vi "TuneFreq.vi"(0 "SG GPIB Address":dbl=22.0, 1 "Trigger Delay":dbl=59.0, 2 "Mod Freq (Hz)":dbl=47.0, 3 "Amplitude (V)":dbl=1.0, 4 "Burst count":dbl=205.0, 5 "PS GPIB Address":string="1", 7 "Poly Coeffs":dbl[](array[numeric]), 9 "Field Set (Oe)":dbl, 11 "VNA GPIB Address":refnum<visa-resource-name>="GPIB0::15::INSTR", 12 "IF Bandwidth":dbl=1000.0, 13 "VNA Points":dbl=1000.0, 14 "VNA Frequency":dbl=10.0, 15 "VNA Power (dBm)":string="-10") -> (8 "Re Freq":dbl format="%.4f")   [LabVIEW 2015]
uses:
  <vilib>/Utility/file.llb/Read Delimited Spreadsheet (DBL).vi
panel:
  out "Im Freq":dbl format="%.4f"
  out "Phase":dbl[][](graph)
  out "Amplitude":dbl[][](graph)
  out "Re phase (deg)":dbl format="%.3f"
  out "Re amplitude":dbl format="%.2e"
  out "Im phase (deg)":dbl format="%.3f"
  out "Im amplitude":dbl format="%.2e"
  out "Im VNA Output":cluster{"X-values":dbl[], "Input data":dbl[]}[](graph)
  out "Re VNA Output":cluster{"X-values":dbl[], "Input data":dbl[]}[](graph)
  in  "Done":bool
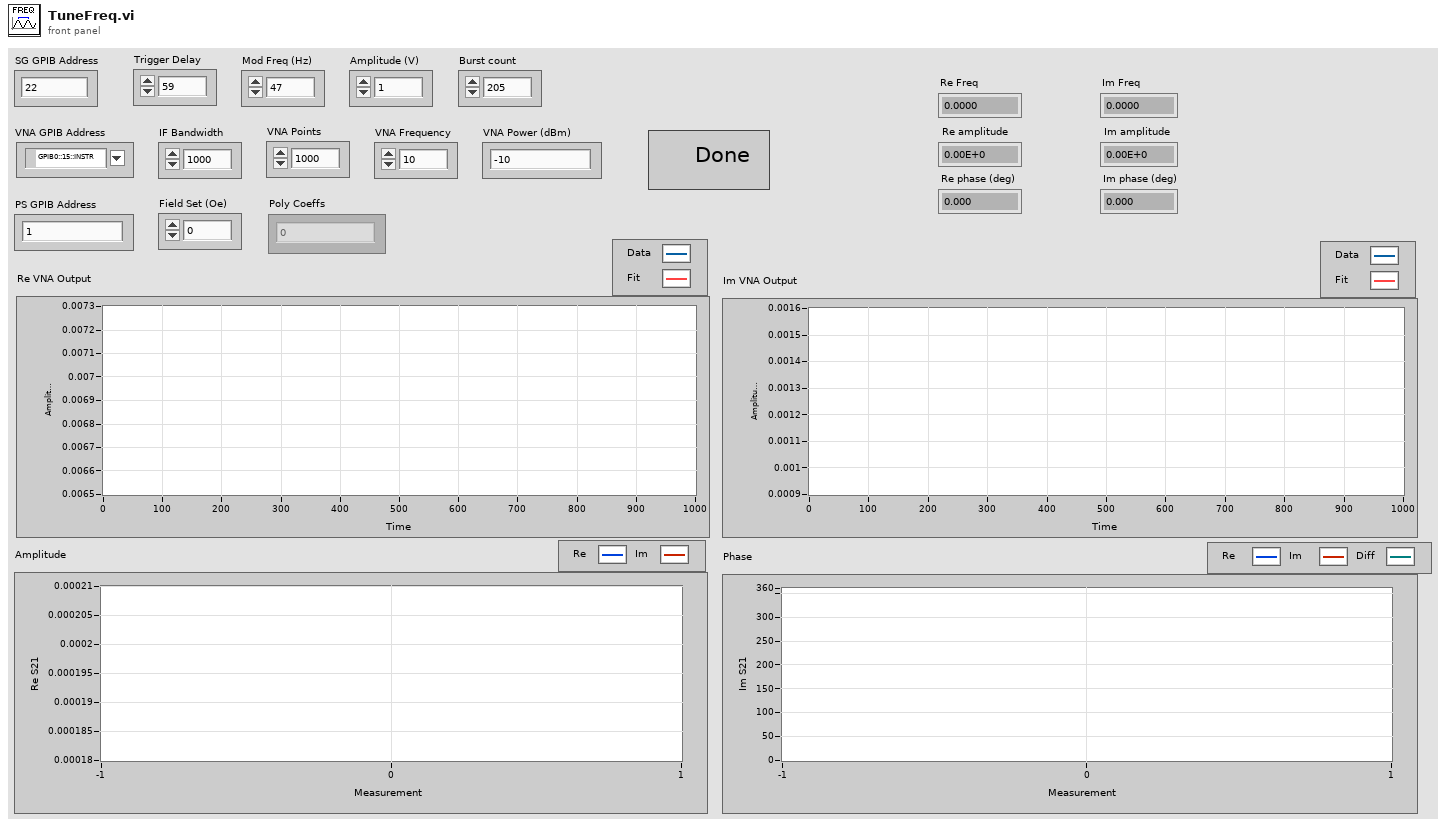
[diagram p1: front panel]
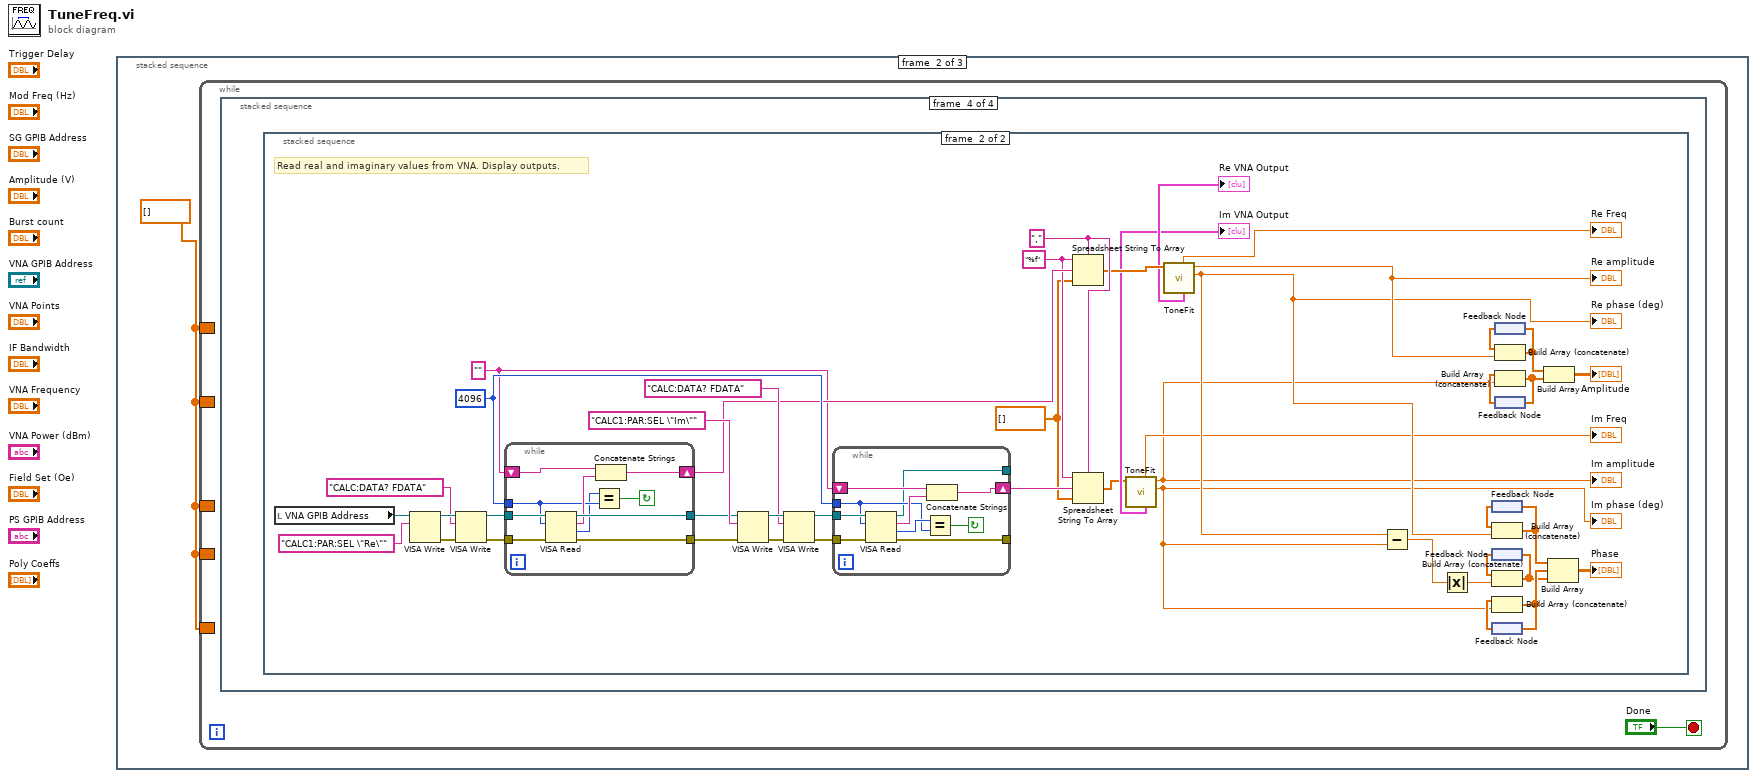
[diagram p0: block diagram]
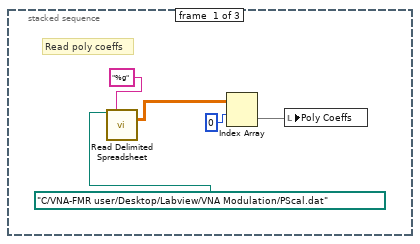
[diagram p2: hidden frame]
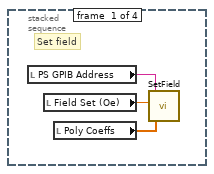
[diagram p3: hidden frame]
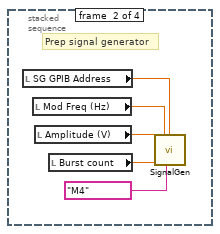
[diagram p4: hidden frame]
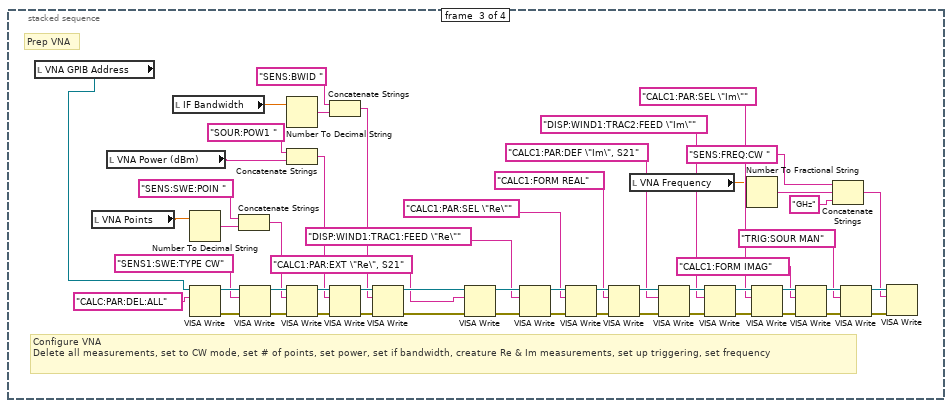
[diagram p5: hidden frame]
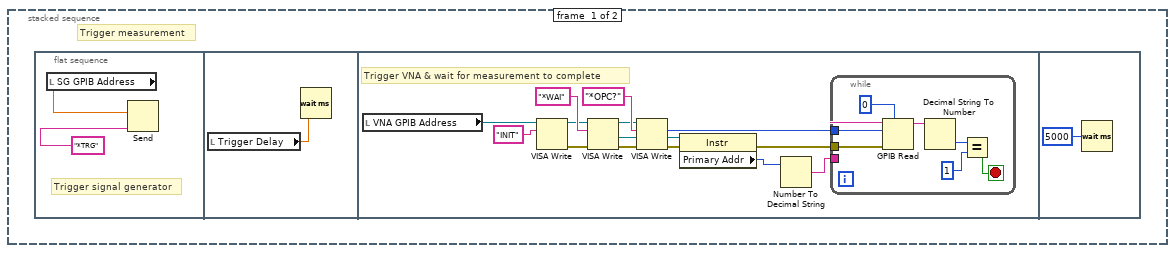
[diagram p6: hidden frame]
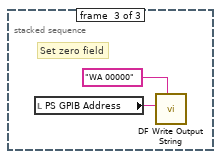
[diagram p7: hidden frame]
diagram:
  n1 = stacked-sequence {
    frame #0 {
      # "Read poly coeffs"
      n2 = call-poly <vilib>:"Read Delimited Spreadsheet.vi"("file path (dialog if empty)"=path "C:/VNA-FMR user/Desktop/Labview/VNA Modulation/PScal.dat", "format (%.3f)"="%g") -> ("all rows"=w3:dbl[][])  [unwired: 8 in, 5 out]
      n3 = Index Array(array=w3, index (row)=0 ("disabled index (col)")) -> (element=w1:dbl[])  [unwired: 1 in]
      n4 = local write "Poly Coeffs"(w1) -> ()
    }
    frame #1 {
      w6 = dbl[] []
      n5 = while {
        border: w6 -> [_]
        border: w6 -> [_]
        border: w6 -> [_]
        border: w6 -> [_]
        border: w6 -> [_]
        stop <- "Done" stop-if-true
        n6 = stacked-sequence {
          frame #0 {
            # "Set field"
            n7 = local read "PS GPIB Address"() -> (w10:string)
            n8 = local read "Field Set (Oe)"() -> (w9:dbl)
            n9 = local read "Poly Coeffs"() -> (w8:dbl[])
            n10 = call "SetField.vi"("Poly Coeffs"=w8, "Field Setpoint"=w9, "PS GPIB Address"=w10) -> ()  [unwired: 9 in]
          }
          frame #1 {
            # "Prep signal generator"
            n11 = local read "SG GPIB Address"() -> (w15:dbl)
            n12 = local read "Mod Freq (Hz)"() -> (w14:dbl)
            n13 = local read "Amplitude (V)"() -> (w13:dbl)
            n14 = local read "Burst count"() -> (w12:dbl)
            n15 = call "SignalGen.vi"("Trigger Mode (Cont)"="M4", "Burst Count"=w12, "Amplitide (V)"=w13, "Modulation Frequency (Hz)"=w14, "SG GPIB Address"=w15) -> ()  [unwired: 7 in]
          }
          frame #2 {
            # "Configure VNA\nDelete all measurements, set to CW mode, set # of points, set power, set if bandwidth, creature Re & Im measurements, set up triggering, set frequency"
            # "Prep VNA"
            n16 = local read "VNA GPIB Address"() -> (w20:refnum<visa-resource-name>)
            n17 = local read "VNA Points"() -> (w19:dbl)
            n18 = local read "VNA Power (dBm)"() -> (w18:string)
            n19 = local read "IF Bandwidth"() -> (w17:dbl)
            n20 = Number To Decimal String(number=w19) -> (decimal integer string=w66:string)  [unwired: 1 in]
            n21 = VISA Write(VISA resource name=w20, write buffer="CALC:PAR:DEL:ALL" ("Characters to Write")) -> (VISA resource name out=w71:refnum<visa-resource-name>, error out=w28:errorcluster)  [unwired: 1 in, 1 out]
            n22 = Concatenate Strings("SENS:SWE:POIN " ("Characters to Write"), w66) -> (w65:string)
            n23 = VISA Write(VISA resource name=w71, write buffer="SENS1:SWE:TYPE CW" ("Characters to Write"), error in (no error)=w28) -> (VISA resource name out=w68:refnum<visa-resource-name>, error out=w69:errorcluster)  [unwired: 1 out]
            n24 = Number To Decimal String(number=w17) -> (decimal integer string=w57:string)  [unwired: 1 in]
            n25 = Concatenate Strings("SOUR:POW1 " ("Characters to Write"), w18) -> (w61:string)
            n26 = VISA Write(VISA resource name=w68, write buffer=w65, error in (no error)=w69) -> (VISA resource name out=w63:refnum<visa-resource-name>, error out=w64:errorcluster)  [unwired: 1 out]
            n27 = Concatenate Strings("SENS:BWID " ("Characters to Write"), w57) -> (w56:string)
            n28 = VISA Write(VISA resource name=w63, write buffer=w61, error in (no error)=w64) -> (VISA resource name out=w59:refnum<visa-resource-name>, error out=w60:errorcluster)  [unwired: 1 out]
            n29 = VISA Write(VISA resource name=w59, write buffer=w56, error in (no error)=w60) -> (VISA resource name out=w54:refnum<visa-resource-name>, error out=w55:errorcluster)  [unwired: 1 out]
            n30 = VISA Write(VISA resource name=w54, write buffer="CALC1:PAR:EXT \"Re\", S21" ("Characters to Write"), error in (no error)=w55) -> (VISA resource name out=w51:refnum<visa-resource-name>, error out=w52:errorcluster)  [unwired: 1 out]
            n31 = VISA Write(VISA resource name=w51, write buffer="DISP:WIND1:TRAC1:FEED \"Re\"" ("Characters to Write"), error in (no error)=w52) -> (VISA resource name out=w48:refnum<visa-resource-name>, error out=w49:errorcluster)  [unwired: 1 out]
            n32 = VISA Write(VISA resource name=w48, write buffer="CALC1:PAR:SEL \"Re\"" ("Characters to Write"), error in (no error)=w49) -> (VISA resource name out=w45:refnum<visa-resource-name>, error out=w46:errorcluster)  [unwired: 1 out]
            n33 = VISA Write(VISA resource name=w45, write buffer="CALC1:FORM REAL" ("Characters to Write"), error in (no error)=w46) -> (VISA resource name out=w42:refnum<visa-resource-name>, error out=w43:errorcluster)  [unwired: 1 out]
            n34 = local read "VNA Frequency"() -> (w16:dbl)
            n35 = VISA Write(VISA resource name=w42, write buffer="CALC1:PAR:DEF \"Im\", S21" ("Characters to Write"), error in (no error)=w43) -> (VISA resource name out=w40:refnum<visa-resource-name>, error out=w39:errorcluster)  [unwired: 1 out]
            n36 = VISA Write(VISA resource name=w40, write buffer="DISP:WIND1:TRAC2:FEED \"Im\"" ("Characters to Write"), error in (no error)=w39) -> (VISA resource name out=w36:refnum<visa-resource-name>, error out=w37:errorcluster)  [unwired: 1 out]
            n37 = Number To Fractional String(number=w16) -> (F-format string=w23:string)  [unwired: 3 in]
            n38 = VISA Write(VISA resource name=w36, write buffer="CALC1:PAR:SEL \"Im\"" ("Characters to Write"), error in (no error)=w37) -> (VISA resource name out=w33:refnum<visa-resource-name>, error out=w34:errorcluster)  [unwired: 1 out]
            n39 = VISA Write(VISA resource name=w33, write buffer="CALC1:FORM IMAG" ("Characters to Write"), error in (no error)=w34) -> (VISA resource name out=w30:refnum<visa-resource-name>, error out=w31:errorcluster)  [unwired: 1 out]
            n40 = Concatenate Strings("SENS:FREQ:CW " ("Characters to Write"), w23, "GHz" ("string")) -> (w21:string)
            n41 = VISA Write(VISA resource name=w30, write buffer="TRIG:SOUR MAN", error in (no error)=w31) -> (VISA resource name out=w25:refnum<visa-resource-name>, error out=w26:errorcluster)  [unwired: 1 out]
            n42 = VISA Write(VISA resource name=w25, write buffer=w21, error in (no error)=w26) -> ()  [unwired: 3 out]
          }
          frame #3 {
            n43 = stacked-sequence {
              frame #0 {
                # "Trigger measurement"
                n44 = flat-sequence {
                  frame #0 {
                    # "Trigger signal generator"
                    n45 = local read "SG GPIB Address"() -> (w73:dbl)
                    n46 = Send(2:w73, 5:"*TRG") -> ()  [unwired: 3 in, 3 out]
                  }
                  frame #1 {
                    n47 = local read "Trigger Delay"() -> (w74:dbl)
                    n48 = Wait (ms)(milliseconds to wait=w74) -> ()  [unwired: 1 out]
                  }
                  frame #2 {
                    # "Trigger VNA & wait for measurement to complete"
                    n49 = local read "VNA GPIB Address"() -> (w87:refnum<visa-resource-name>)
                    n50 = VISA Write(VISA resource name=w87, write buffer="INIT") -> (VISA resource name out=w85:refnum<visa-resource-name>, error out=w84:errorcluster)  [unwired: 1 in, 1 out]
                    n51 = VISA Write(VISA resource name=w85, write buffer="*WAI", error in (no error)=w84) -> (VISA resource name out=w75:refnum<visa-resource-name>, error out=w82:errorcluster)  [unwired: 1 out]
                    n52 = VISA Write(VISA resource name=w75, write buffer="*OPC?", error in (no error)=w82) -> (VISA resource name out=w79:refnum<visa-resource-name>, return count=w81:u32, error out=w78:errorcluster)
                    n53 = property class="Instr"(reference=w79, error in=w78) -> (error out=w77:errorcluster, "Primary Addr"=w76:u16)  [unwired: 1 out]
                    n54 = Number To Decimal String(number=w76) -> (decimal integer string=w80:string)  [unwired: 1 in]
                    n55 = while {
                      tunnel: w77 -> [w92]
                      tunnel: w81 -> [w91]
                      tunnel: w80 -> [w89]
                      stop <- w94 stop-if-true
                      n56 = GPIB Read(0:w89, 1:w91, 3:w92, 4:0 ("timeout ms (488.2 global)")) -> (5:w93:string)  [unwired: 1 in, 2 out]
                      n57 = Decimal String To Number(string=w93) -> (number=w96:i32)  [unwired: 2 in, 1 out]
                      n58 = Equal?(x=w96, y=1) -> (x = y?=w94:bool)
                    }
                  }
                  frame #3 {
                    n59 = Wait (ms)(milliseconds to wait=u32 5000) -> ()  [unwired: 1 out]
                  }
                }
              }
              frame #1 {
                w122 = ""
                w125 = dbl[] [] ("X")
                w126 = "%f" ("format string")
                w127 = "," ("delimiter (Tab)")
                w131 = 4096
                # "Read real and imaginary values from VNA. Display outputs."
                n60 = local read "VNA GPIB Address"() -> (w130:refnum<visa-resource-name>)
                n61 = VISA Write(VISA resource name=w130, write buffer="CALC1:PAR:SEL \"Re\"" ("Characters to Write")) -> (VISA resource name out=w141:refnum<visa-resource-name>, error out=w142:errorcluster)  [unwired: 1 in, 1 out]
                n62 = VISA Write(VISA resource name=w141, write buffer="CALC:DATA? FDATA", error in (no error)=w142) -> (VISA resource name out=w139:refnum<visa-resource-name>, error out=w138:errorcluster)  [unwired: 1 out]
                n63 = while {
                  tunnel: w131 -> [w155]
                  tunnel: w139 -> [w163]
                  tunnel: [w160] -> w123
                  tunnel: w138 -> [w162]
                  tunnel: [w161] -> w124
                  shift-right: [w156] -> w129
                  shift-left: w122 -> [w157]
                  stop <- w159 continue-if-true
                  n64 = VISA Read(VISA resource name=w163, byte count=w155, error in (no error)=w162) -> (VISA resource name out=w160:refnum<visa-resource-name>, read buffer=w158:string, return count=w154:u32, error out=w161:errorcluster)
                  n65 = Equal?(x=w154, y=w155) -> (x = y?=w159:bool)
                  n66 = Concatenate Strings(w157, w158) -> (w156:string)
                }
                n67 = VISA Write(VISA resource name=w123, write buffer="CALC1:PAR:SEL \"Im\"" ("Characters to Write"), error in (no error)=w124) -> (VISA resource name out=w135:refnum<visa-resource-name>, error out=w136:errorcluster)  [unwired: 1 out]
                n68 = VISA Write(VISA resource name=w135, write buffer="CALC:DATA? FDATA", error in (no error)=w136) -> (VISA resource name out=w133:refnum<visa-resource-name>, error out=w132:errorcluster)  [unwired: 1 out]
                n69 = while {
                  tunnel: w133 -> [w153]
                  tunnel: w132 -> [w152]
                  tunnel: w131 -> [w147]
                  shift-right: [w150] -> w128
                  shift-left: w122 -> [w149]
                  tunnel: [w145] -> _
                  tunnel: [w144] -> _
                  stop <- w146 continue-if-true
                  n70 = VISA Read(VISA resource name=w153, byte count=w147, error in (no error)=w152) -> (VISA resource name out=w145:refnum<visa-resource-name>, read buffer=w151:string, return count=w148:u32, error out=w144:errorcluster)
                  n71 = Equal?(x=w148, y=w147) -> (x = y?=w146:bool)
                  n72 = Concatenate Strings(w149, w151) -> (w150:string)
                }
                n73 = Spreadsheet String To Array(delimiter (Tab)=w127, format string=w126, spreadsheet string=w129, array type (2D Dbl)=w125) -> (array=w101:dbl[])
                n74 = Spreadsheet String To Array(delimiter (Tab)=w127, format string=w126, spreadsheet string=w128, array type (2D Dbl)=w125) -> (array=w98:dbl[])
                n75 = call "ToneFit.vi"("Input data"=w98) -> ("Phase"=w102:dbl, "Amplitude"=w103:dbl, "XY Graph"=→"Im VNA Output":cluster{"X-values":dbl[], "Input data":dbl[]}[], "Frequency"=→"Im Freq":dbl)  [unwired: 7 in]
                "Im amplitude" <- w103
                "Im phase (deg)" <- w102
                n76 = call "ToneFit.vi"("Input data"=w101) -> ("Phase"=w105:dbl, "Amplitude"=w106:dbl, "XY Graph"=→"Re VNA Output":cluster{"X-values":dbl[], "Input data":dbl[]}[], "Frequency"=→"Re Freq":dbl)  [unwired: 7 in]
                "Re amplitude" <- w106
                "Re phase (deg)" <- w105
                n77 = Subtract(x=w105, y=w102) -> (x-y=w111:dbl)
                n78 = Absolute Value(x=w111) -> (abs(x)=w110:dbl)
                n79 = feedback #1() -> (w120:dbl[])
                n80 = Build Array (concatenate)(w120, w105) -> (w114:dbl[])
                n81 = feedback-in #1(w114) -> ()
                n82 = feedback #2() -> (w109:dbl[])
                n83 = Build Array (concatenate)(w109, w110) -> (w108:dbl[])
                n84 = feedback-in #2(w108) -> ()
                n85 = feedback #3() -> (w118:dbl[])
                n86 = Build Array (concatenate)(w118, w102) -> (w113:dbl[])
                n87 = feedback-in #3(w113) -> ()
                n88 = feedback #4() -> (w121:dbl[])
                n89 = Build Array (concatenate)(w121, w106) -> (w116:dbl[])
                n90 = feedback-in #4(w116) -> ()
                n91 = feedback #5() -> (w119:dbl[])
                n92 = Build Array (concatenate)(w119, w103) -> (w117:dbl[])
                n93 = feedback-in #5(w117) -> ()
                n94 = Build Array(w116, w117) -> (→"Amplitude":dbl[][])
                n95 = Build Array(w114, w113, w108) -> (→"Phase":dbl[][])
              }
            }
          }
        }
      }
    }
    frame #2 {
      # "Set zero field"
      n96 = local read "PS GPIB Address"() -> (w165:string)
      n97 = call "DF Write Output String"("Write String"="WA 00000", "GPIB Address"=w165) -> ()  [unwired: 7 in]
    }
  }
